vi "rename file.vi"(8 "error in":errorcluster, 10 "Starting Number":i32, 11 "path":path) -> (0 "error out":errorcluster)   [LabVIEW 2023]
panel:
  out "deleted portion":string
  out "Array":string[](array[string])
  out "created path":path
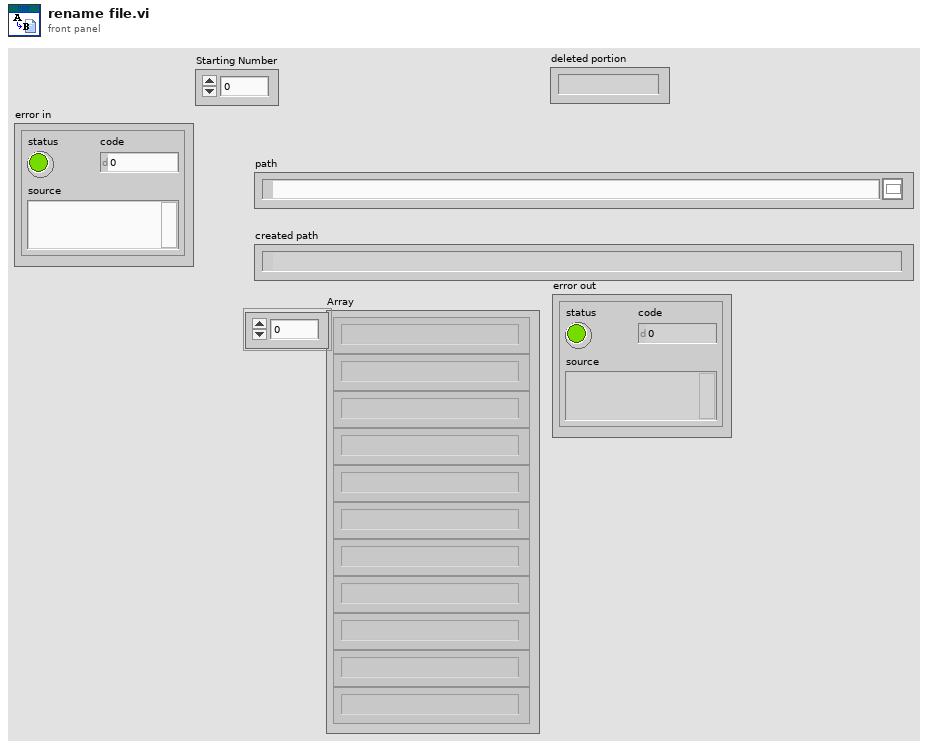
[diagram p1: front panel]
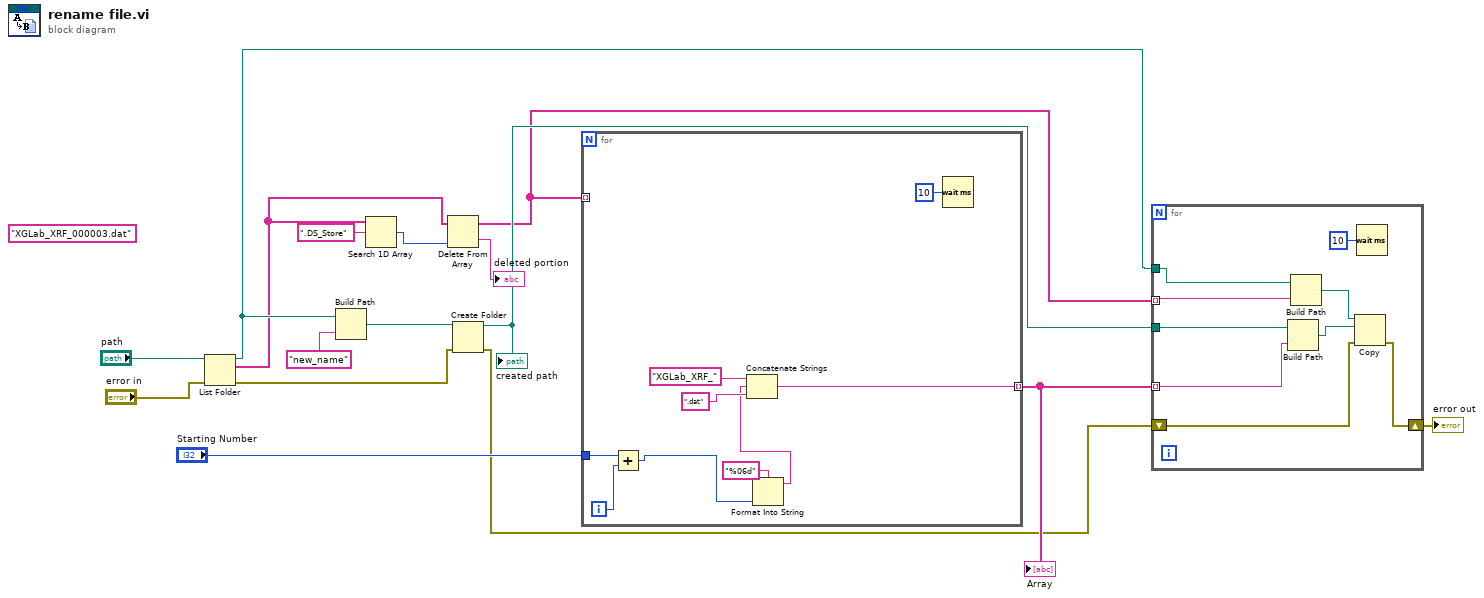
[diagram p0: block diagram]
diagram:
  (unwired) "XGLab_XRF_000003.dat"
  n1 = List Folder(path="path", error in="error in") -> (path out=w12:path, filenames=w3:string[], error out=w8:errorcluster)  [unwired: 2 in, 1 out]
  n2 = Build Path(base path=w12, name or relative path="new_name" ("prompt (Create Folder)")) -> (appended path=w13:path)
  n3 = Search 1D Array(1D array=w3, element=".DS_Store") -> (index of element=w4:i32)  [unwired: 1 in]
  n4 = Delete From Array(array=w3, index=w4) -> (deleted portion=→"deleted portion":string, array with subset deleted=w2:string[])  [unwired: 1 in]
  n5 = Create Folder(path (use dialog)=w13, error in=w8) -> (created path=w11:path, error out=w7:errorcluster)  [unwired: 1 in, 1 out]
  "created path" <- w11
  n6 = for {
    tunnel: w2 -> [_] mode=indexing
    tunnel: [w18] -> w10 mode=indexing
    tunnel: "Starting Number" -> [w17]
    i -> [w25]
    n7 = Add(x=w17, y=w25) -> (x+y=w24:i32)
    n8 = Format Into String(format string="%06d", w24) -> (resulting string=w20:string)  [unwired: 2 in, 1 out]
    n9 = Concatenate Strings("XGLab_XRF_" ("regular expression"), w20, ".dat" ("regular expression")) -> (w18:string)
    n10 = Wait (ms)(milliseconds to wait=u32 10) -> ()  [unwired: 1 out]
  }
  "Array" <- w10
  n11 = for {
    tunnel: w2 -> [w32] mode=indexing
    tunnel: w12 -> [w33]
    tunnel: w11 -> [w30]
    tunnel: w10 -> [w29] mode=indexing
    shift-right: [w26] -> w6
    shift-left: w7 -> [w27]
    n12 = Build Path(base path=w30, name or relative path=w29) -> (appended path=w28:path)
    n13 = Build Path(base path=w33, name or relative path=w32) -> (appended path=w34:path)
    n14 = Copy(8:w27, 10:w28, 11:w34) -> (0:w26:errorcluster)  [unwired: 2 in, 2 out]
    n15 = Wait (ms)(milliseconds to wait=u32 10) -> ()  [unwired: 1 out]
  }
  "error out" <- w6
